vi "ConsumerData.vi"(5 "Day of Year":u32, 6 "Unique Object Identifier":string, 7 "Day Time":u32, 8 "Error In":errorcluster, 10 "Energy flow IN":T5, 11 "DataFlowIN":T4) -> (0 "Error Out":errorcluster, 2 "Energy flow OUT":T5, 3 "DataFlowOUT":T4)   [LabVIEW 2017]
uses:
  classes/DataCollector.lvclass
  classes/DataHandler.lvclass
  classes/SimulationParameter.lvclass
panel:
  in  "Operating Parameter":T1
  out "Simulation Parameter":T2
  out "Control Parameter":T3
  out "List of Fieldelements":string[](array[string])
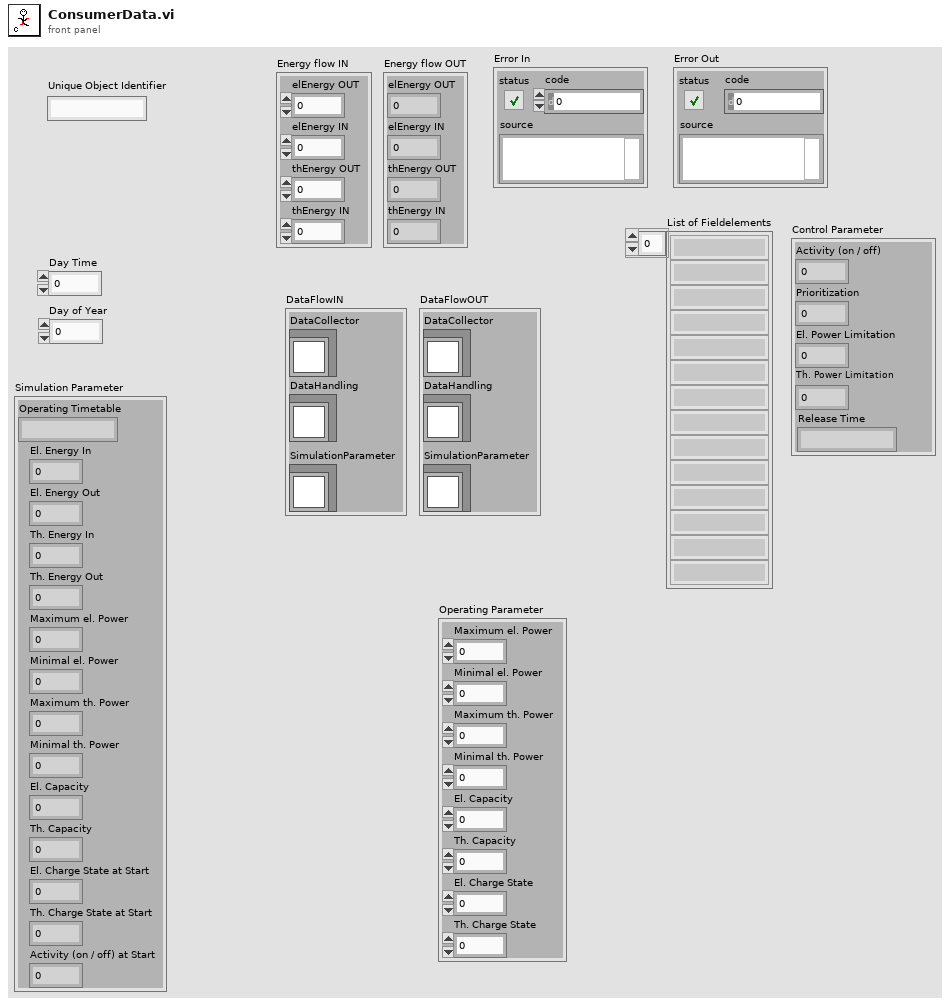
[diagram p1: front panel]
types:
  T1 = cluster{"Maximum el. Power":dbl, "Minimal el. Power":dbl, "Maximum th. Power":dbl, "Minimal th. Power":dbl, "El. Capacity":dbl, "Th. Capacity":dbl, "El. Charge State":dbl, "Th. Charge State":dbl}
  T2 = cluster{"Operating Timetable":string, "El. Energy In":dbl, "El. Energy Out":dbl, "Th. Energy In":dbl, "Th. Energy Out":dbl, "Maximum el. Power":dbl, "Minimal el. Power":dbl, "Maximum th. Power":dbl, "Minimal th. Power":dbl, "El. Capacity":dbl, "Th. Capacity":dbl, "El. Charge State at Start":dbl, "Th. Charge State at Start":dbl, "Activity (on / off) at Start":i64}
  T3 = cluster{"Activity (on / off)":i64, "Prioritization":i64, "El. Power Limitation":dbl, "Th. Power Limitation":dbl, "Release Time":string}
  T4 = cluster{"DataCollector":refnum<class "DataCollector.lvclass">, "DataHandling":refnum<class "DataHandler.lvclass">, "SimulationParameter":refnum<class "SimulationParameter.lvclass">}
  T5 = cluster{"elEnergy OUT":dbl, "elEnergy IN":dbl, "thEnergy OUT":dbl, "thEnergy IN":dbl}
  T6 = cluster{"Day Time":u32, "Day of Year":u32, "Energy flow IN":cluster{"elEnergy OUT":dbl, "elEnergy IN":dbl, "thEnergy OUT":dbl, "thEnergy IN":dbl}, "Operating Parameter":cluster{"Maximum el. Power":dbl, "Minimal el. Power":dbl, "Maximum th. Power":dbl, "Minimal th. Power":dbl, "El. Capacity":dbl, "Th. Capacity":dbl, "El. Charge State":dbl, "Th. Charge State":dbl}, "Control Parameter":cluster{"Activity (on / off)":i64, "Prioritization":i64, "El. Power Limitation":dbl, "Th. Power Limitation":dbl, "Release Time":string}}
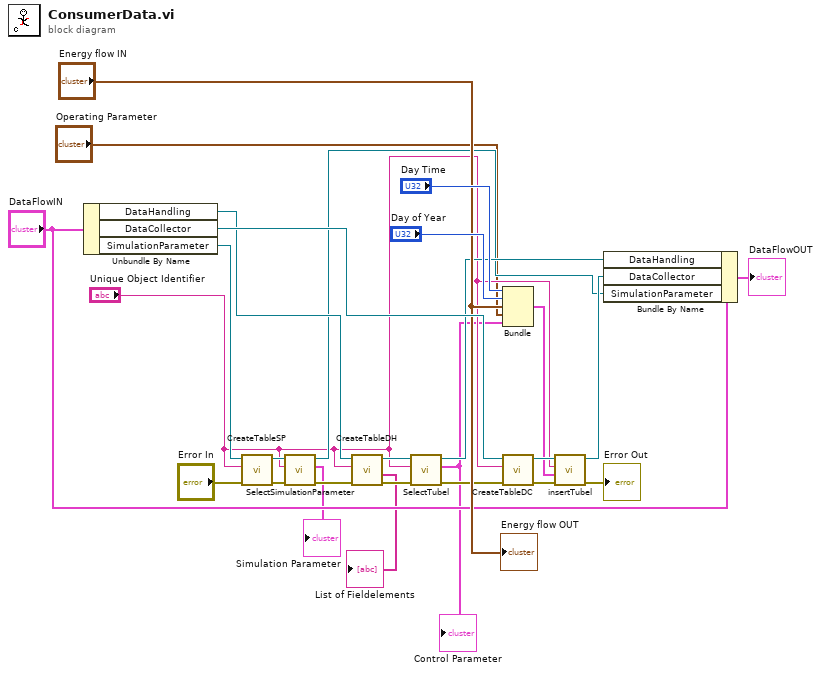
[diagram p0: block diagram]
diagram:
  n1 = Unbundle By Name("DataFlowIN") -> ("DataHandling"=w17:refnum<class "DataHandler.lvclass">, "DataCollector"=w27:refnum<class "DataCollector.lvclass">, "SimulationParameter"=w9:refnum<class "SimulationParameter.lvclass">)
  n2 = call-dynamic "CreateTableSP.vi"("error in (no error)"="Error In", "Name of Table"="Unique Object Identifier", "SimulationParameter in"=w9) -> ("error out"=w8:errorcluster, "SimulationParameter out"=w7:refnum<class "SimulationParameter.lvclass">)  [unwired: 5 in, 2 out]
  n3 = call-dynamic "SelectSimulationParameter.vi"("error in (no error)"=w8, "Unique Object Identifier"="Unique Object Identifier", "SimulationParameter in"=w7) -> ("error out"=w5:errorcluster, "Cluster"=→"Simulation Parameter":T2, "SimulationParameter out"=w6:refnum<class "SimulationParameter.lvclass">)  [unwired: 6 in]
  n4 = call-dynamic "CreateTableDH.vi"("error in (no error)"=w5, "Name of Table"="Unique Object Identifier", "DataHandler in"=w17) -> ("error out"=w14:errorcluster, "List of Fieldelements"=→"List of Fieldelements":string[], "DataHandler out"=w16:refnum<class "DataHandler.lvclass">)  [unwired: 5 in, 1 out]
  n5 = call-dynamic "SelectTubel.vi"("error in (no error)"=w14, "Unique Object Identifier"="Unique Object Identifier", "DataHandler in"=w16) -> ("error out"=w13:errorcluster, "Control Parameter"=w1:T3, "DataHandler out"=w15:refnum<class "DataHandler.lvclass">)  [unwired: 6 in]
  "Control Parameter" <- w1
  n6 = Bundle("Day Time"="Day Time", "Day of Year"="Day of Year", "Energy flow IN"="Energy flow IN", "Operating Parameter"="Operating Parameter", "Control Parameter"=w1) -> (w12:T6)  [unwired: 1 in]
  n7 = call "CreateTableDC.vi"("error in (no error)"=w13, "Name of Table"="Unique Object Identifier", "DataCollector in"=w27) -> ("error out"=w26:errorcluster, "DataCollector out"=w24:refnum<class "DataCollector.lvclass">)  [unwired: 7 in]
  n8 = call-dynamic "insertTubel.vi"("error in (no error)"=w26, "Data Cluster"=w12, "Name of Table"="Unique Object Identifier", "DataCollector in"=w24) -> ("error out"=→"Error Out":errorcluster, "DataCollector out"=w23:refnum<class "DataCollector.lvclass">)  [unwired: 6 in]
  n9 = Bundle By Name(cluster="DataFlowIN", "DataHandling"=w15, "DataCollector"=w23, "SimulationParameter"=w6) -> (→"DataFlowOUT":T4)
  "Energy flow OUT" <- "Energy flow IN"
